vi "Text control 2 v0.5.vi"() -> ()   [LabVIEW 2016]
panel:
  out "error out":errorcluster
  in  "Units":bool
  out "Elapsed Time":dbl caption="Elapsed Time (s)"
  out "Ion vs time":cluster{"Y data in":dbl[], "X data in":dbl[]}[](graph)
  out "Ig":dbl format="%.2e"
  out "Id":dbl format="%.2e"
  out "Is":dbl format="%.2e"
  out "I vs Vg":cluster{"Y data in":dbl[], "X data in":dbl[]}[](graph)
  in  "Panel Controls 2":T1={"Emergency Stop"=refnum, "TransGraph Max"=1e-05, "Text/Graph (text=false)"=TRUE, "TransGraph Min"=1e-11} {"TransGraph Min" format="%.2e"; "TransGraph Max" format="%.2e"}
  out "Currently running:":string="#output s 0 0 0 -0.008 0.008 0.002"
  in  "Lines left to run:":string
  in  "Standby":T2
  in  "Full Reset":bool
  in  "SMU4":cluster{"on/off":bool, "Voltage":dbl} {"Voltage" min=-100.0 max=100.0 format="%.2f"}
  in  "Source/Drain Range":u8(slide)=6 max=11 scale=0.0..11.0
  in  "Source/Drain\nRange mode":u16(ring) items=["Auto", "Limited", "Fixed"]
  in  "Gate Range":u8(slide)=6 max=11 scale=0.0..11.0
  in  "Gate Range\nmode":u16(ring) items=["Auto", "Limited", "Fixed"]
  in  "Gate":T3={"Gate Start"=0.0, "Gate Stop"=2.0, "Gate Step (linear only)"=1.0, "Gate Compliance"=0.0001, "Gate PComp"=0.0, "Range mode"=0, "Range"=6} {"Range" max=11 scale=0.0..11.0; "Range mode" items=["Auto", "Limited", "Fixed"]; "Gate PComp" format="%^.2e"; "Gate Compliance" format="%^.2e"; "Gate Step (linear only)" format="%^.4e"; "Gate Stop" format="%^.4e"; "Gate Start" format="%^.4e"}
  in  "Drain 2":T4={"Drain Start"=0.0, "Drain Stop"=2.0, "Drain Compliance"=0.0001, "Drain Step"=1.0, "Drain PComp"=0.0, "Range mode"=0, "Range"=6} {"Range" max=11 scale=0.0..11.0; "Range mode" items=["Auto", "Limited", "Fixed"]; "Drain PComp" format="%^.2e"; "Drain Step" format="%^.4e"; "Drain Compliance" format="%^.2e"; "Drain Stop" format="%^.4e"; "Drain Start" format="%^.4e"}
  in  "Timings 2":T5={"integration time"=0, "Short/Long integration time"=0.00064, "hold time (sec)"=0.0, "delay time (sec)"=0.0, "Step Time (0 disables)"=0.0, "sweep method"=0, "Pulse period"=0.005, "Base voltage"=0.0, "Pulse width"=0.0005} {"Pulse width" min=0.0005 max=0.1 step=0.0001 format="%.4f"; "Base voltage" format="%^.4e"; "Pulse period" min=0.005 max=1.0 step=0.0001 format="%.4f"; "sweep method" items=["Continuous", "Pulsed"]; "Step Time (0 disables)" format="%.2f"; "delay time (sec)" format="%.4f"; "hold time (sec)" format="%.4f"; "Short/Long integration time" format="%^.0e"; "integration time" scale=0.0..2.0}
  in  "Panel Controls":T6={"Emergency Stop"=refnum, "TransGraph Max"=1e-05, "Text/Graph (text=false)"=TRUE} {"TransGraph Max" format="%.2e"}
  in  "Interrupt run":bool
  in  "Drain: Compliance":dbl=0.001 format="%.8f"
  in  "Gate: Compliance":dbl=0.001 format="%.8f"
  out "Path":path=path "C:/users/rlp38/09Apr2009LTtesting/test2.txt"
  in  "hold time /s":dbl format="%.2f"
  in  "delay time /s":dbl format="%.2f"
  in  "integration time":u32(slide) max=2 step=1 scale=0.0..2.0
  in  "Integration time (short)":dbl=0.0019 min=8e-05 max=0.0019 step=8e-05 format="%^.0e"
  in  "Integration time (long)":dbl=0.32 min=0.04 max=2.0 step=0.02 format="%.2f"
  in  "Step delay /s":dbl format="%.2f"
  in  "Program":string="#pulsedstressV d 0.03 20 0 0.5 0.0827 5\n#\nitime s\ngaterangemode l\ndrainrangemode l\n#pulsed on 0.05 0 0.02\ntransfer d 1 -1 -0.1 -1 -1 0\nwait-min 1\ntransfer d 1 -1 -0.1 -1 -1 0\n#transfer d -10 40 1 5 40 35\n#transfer d -10 40 1 5 40 35\n#output d 0 40 20 0 40 1\n#\n#\n#sample 1 0.008 221 6 0.003\n#samplei 400e-6 200 6 0.002 0.1\n#vsu2pulse -10 4\n#\n#stressV 0.016 0.03 2e-4 0.1e-3 11\n#stressI 220e-7 0.08 15\n#transfer s -1 1 0.5 -0.005 0.005 0.005\n#output s 0 0 0 -0.008 0.008 0.002\n"
  # "Syntax:\nitime [s|m|l]\ngaterangemode [a|l|f]\ndrainrangemode [a|l|f]\npulsed [on|off] PulsePeriod(sec) PulseBaseVoltage PulseONWidth(sec)\nstandby [on l off]\nwait NumMilliseconds\nwait-min NumMinutes\n# texthere = comment\ntransfer [s|d] VgStart VgStop VgStep VdStart VdStop VdStep\noutput [s|d] VgStart VgStop VgStep VdStart VdStop VdStep\nsample Vg Vd NumSamples Time(s) SampleInterval(s)\nsamplei Idg NumSamples Time(s) SampleInterval(s) VDGcompliance\n# if in doubt use SampleInterval(s) = 0.004\nstressV VG VD IGcompliance IDcompliance Duration(sec)\nstressI IDG VDGcompliance Duration(sec)\nvsu2pulse Bias Duration(s)\npulsedstressV [s|d] VEstop VgON VgOFF Period(s) PulseONwidth(s) Vd\nsample-fpp Vg Vd NumSamples Time\nresample-fpp Vg Vd\ntransfer-fpp [s|d] VgStart VgStop VgStep VdStart VdStop VdStep\noutput-fpp [s|d] VgStart VgStop VgStep VdStart VdStop VdStep"
  # "Sec"
  # "Min"
  # "Original Filename (.txt is removed)-Prefix-ElapsedTime (in sec)-Suffix (must include .txt)"
  # "100 samples is approx 13s with medium integration"
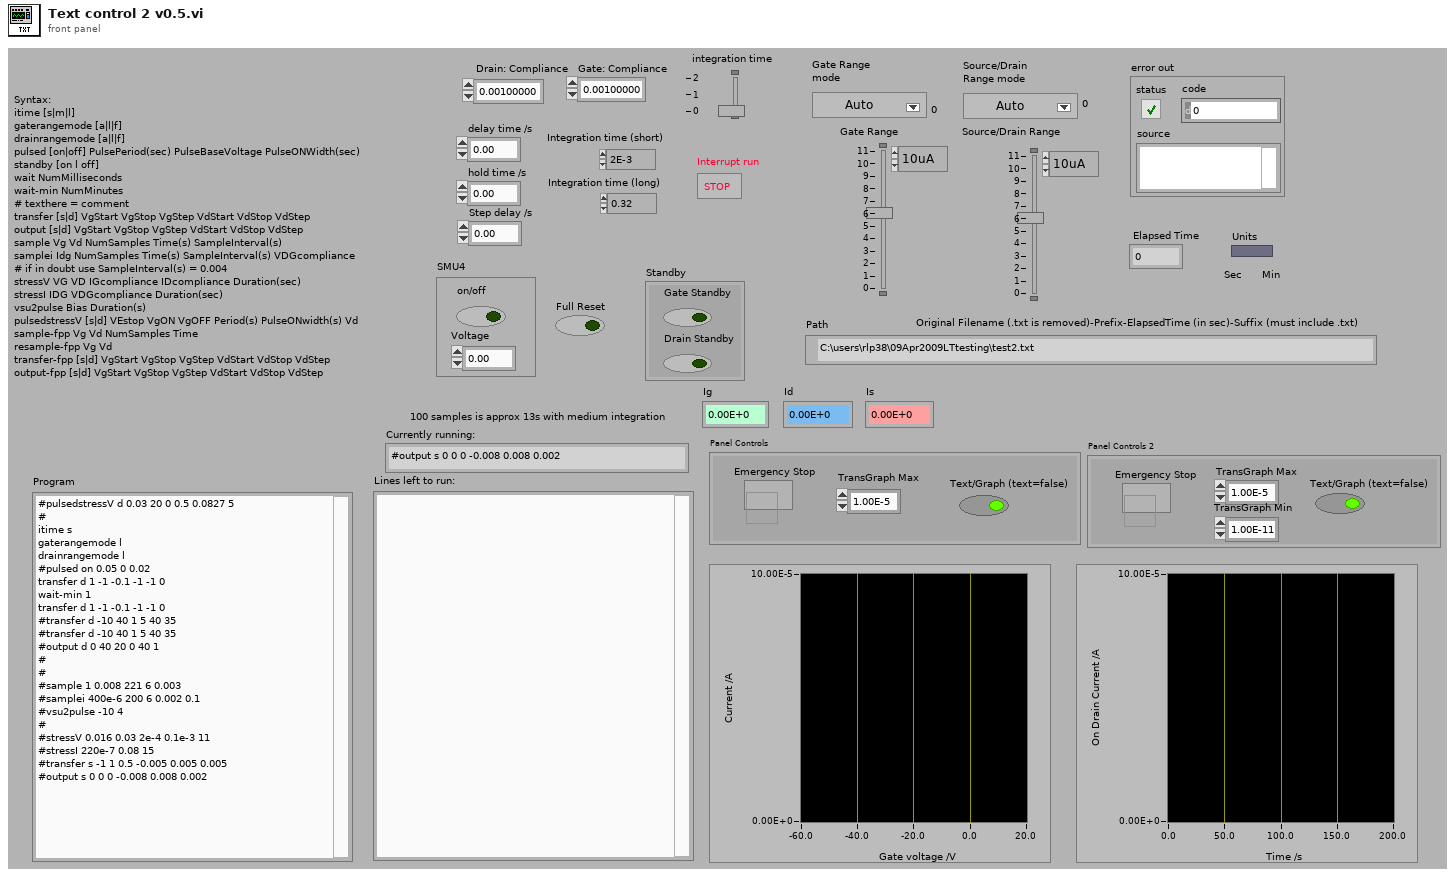
[diagram p1: front panel]
types:
  T1 = cluster{"Emergency Stop":refnum<vi>, "TransGraph Max":dbl, "Text/Graph (text=false)":bool, "TransGraph Min":dbl}
  T2 = cluster{"Gate Standby":bool, "Drain Standby":bool}
  T3 = cluster{"Gate Start":dbl, "Gate Stop":dbl, "Gate Step (linear only)":dbl, "Gate Compliance":dbl, "Gate PComp":dbl, "Range mode":u16, "Range":u8}
  T4 = cluster{"Drain Start":dbl, "Drain Stop":dbl, "Drain Compliance":dbl, "Drain Step":dbl, "Drain PComp":dbl, "Range mode":u16, "Range":u8}
  T5 = cluster{"integration time":u32, "Short/Long integration time":dbl, "hold time (sec)":dbl, "delay time (sec)":dbl, "Step Time (0 disables)":dbl, "sweep method":u16, "Pulse period":dbl, "Base voltage":dbl, "Pulse width":dbl}
  T6 = cluster{"Emergency Stop":refnum<vi>, "TransGraph Max":dbl, "Text/Graph (text=false)":bool}
  T7 = enum16{"open", "replace", "create", "open or create", "replace or create", "replace or create with confirmation"}
  T8 = cluster{"V2 Start":dbl, "V2 Step":dbl, "Number of points":i32}
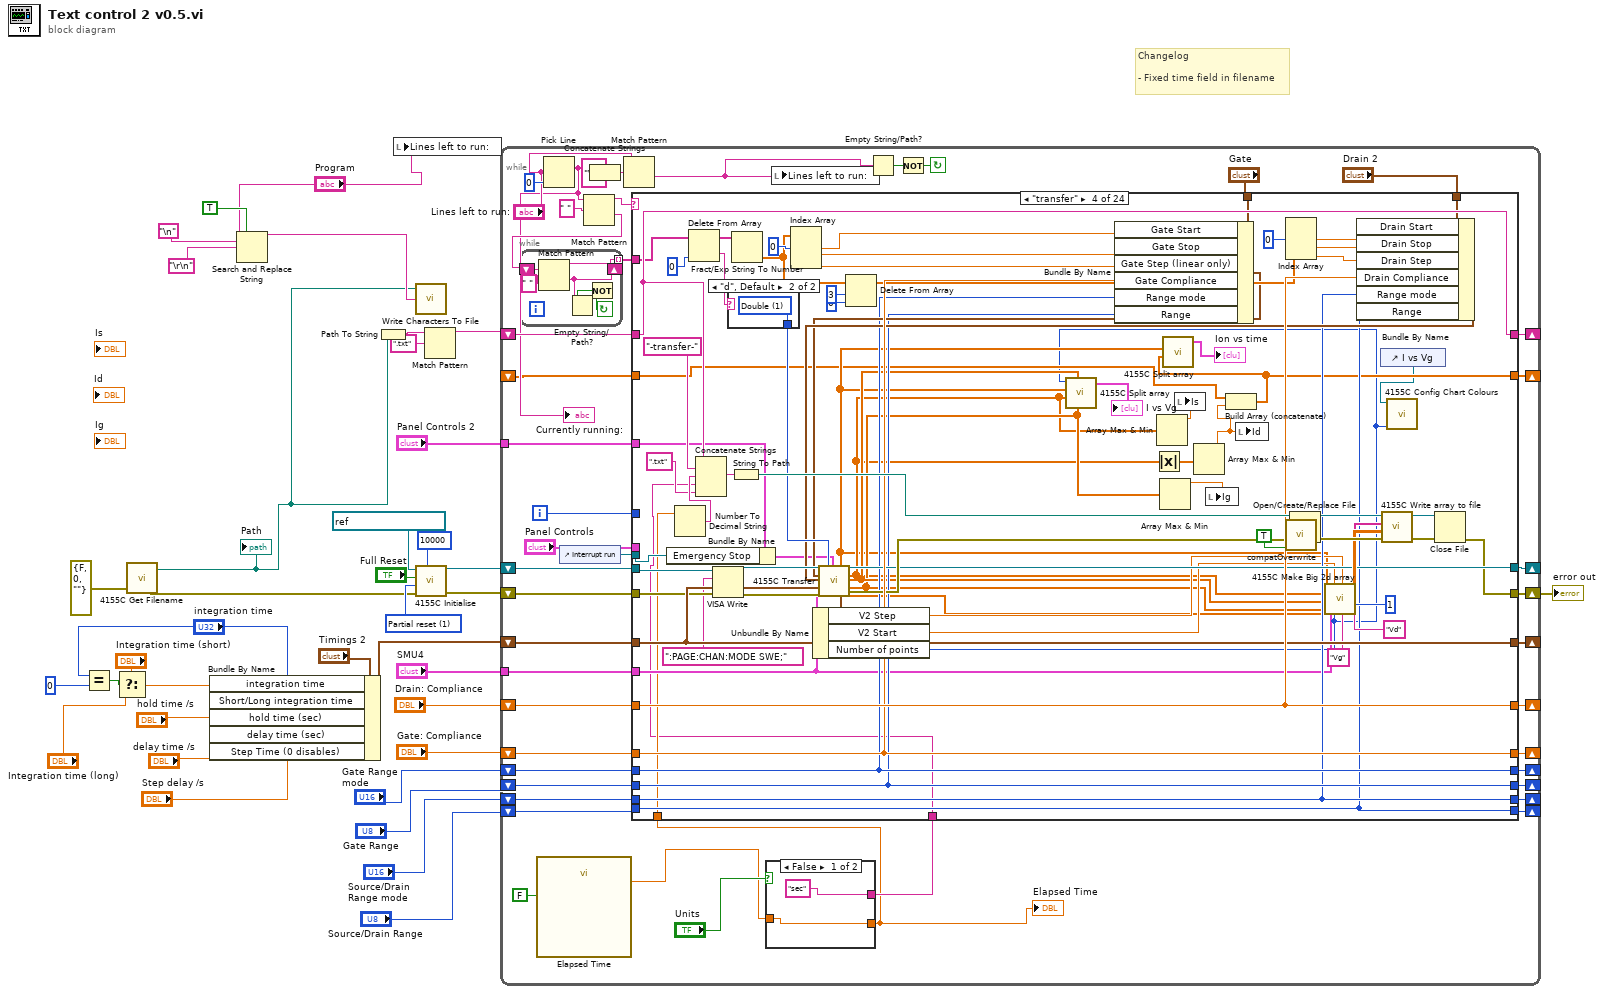
[diagram p0: block diagram]
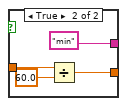
[diagram p2: hidden frame]
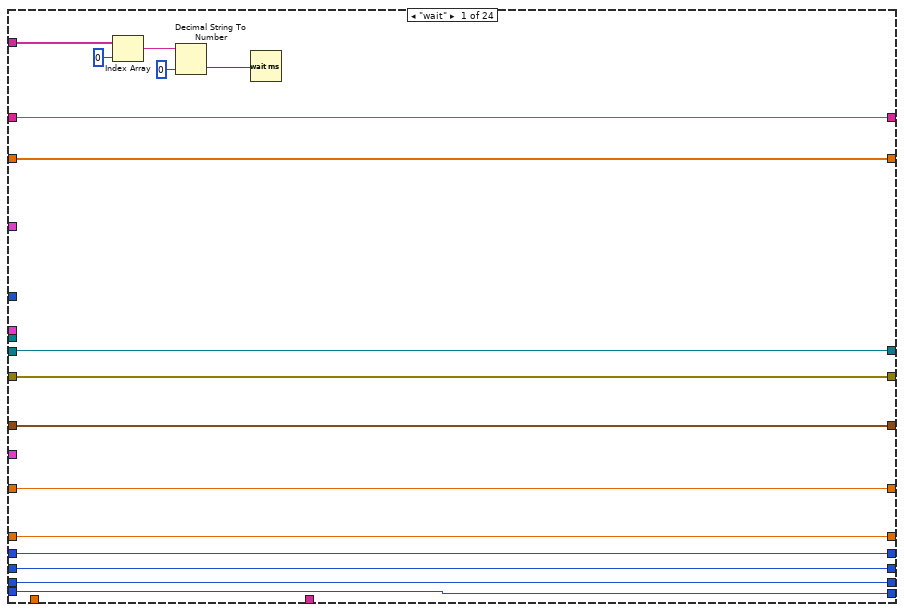
[diagram p3: hidden frame]
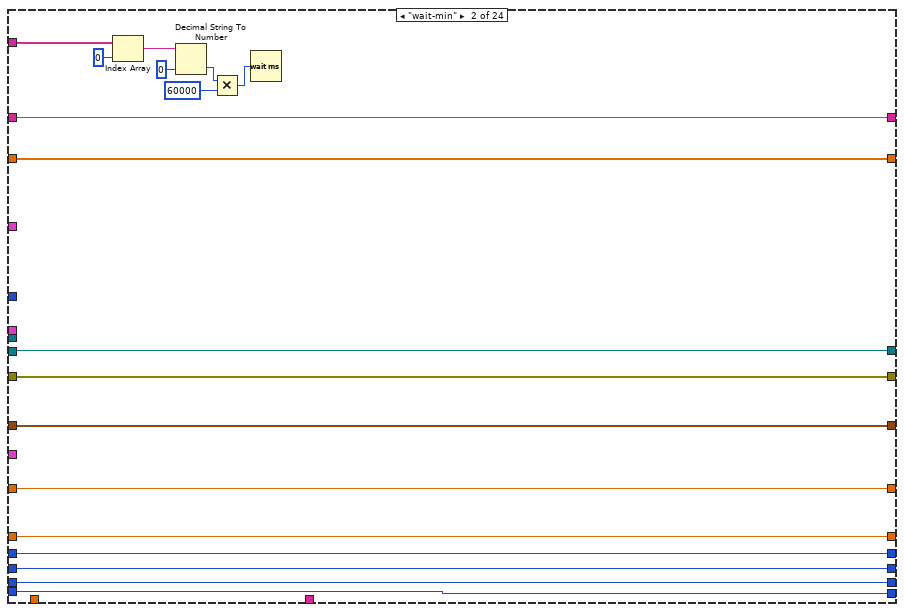
[diagram p4: hidden frame]
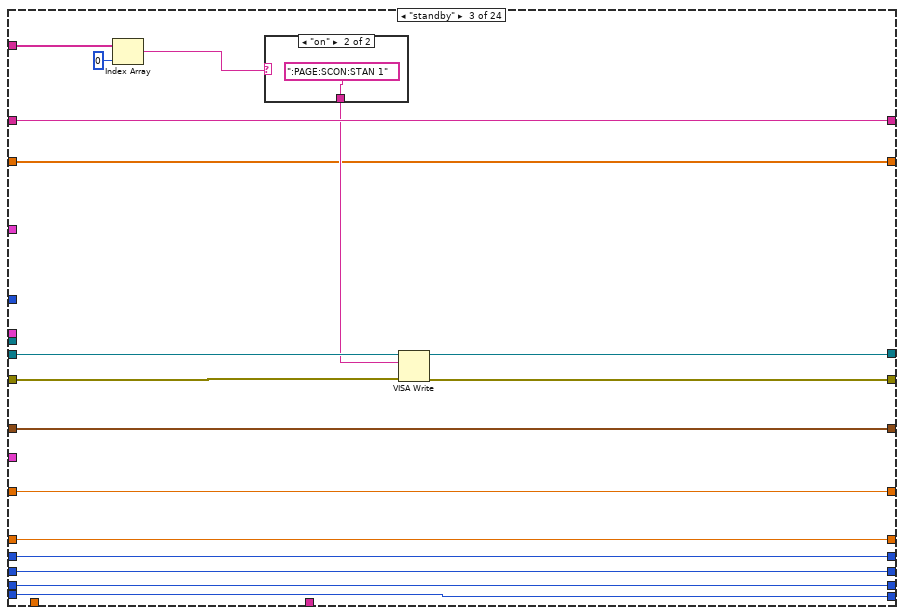
[diagram p5: hidden frame]
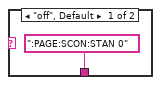
[diagram p6: hidden frame]
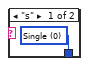
[diagram p7: hidden frame]
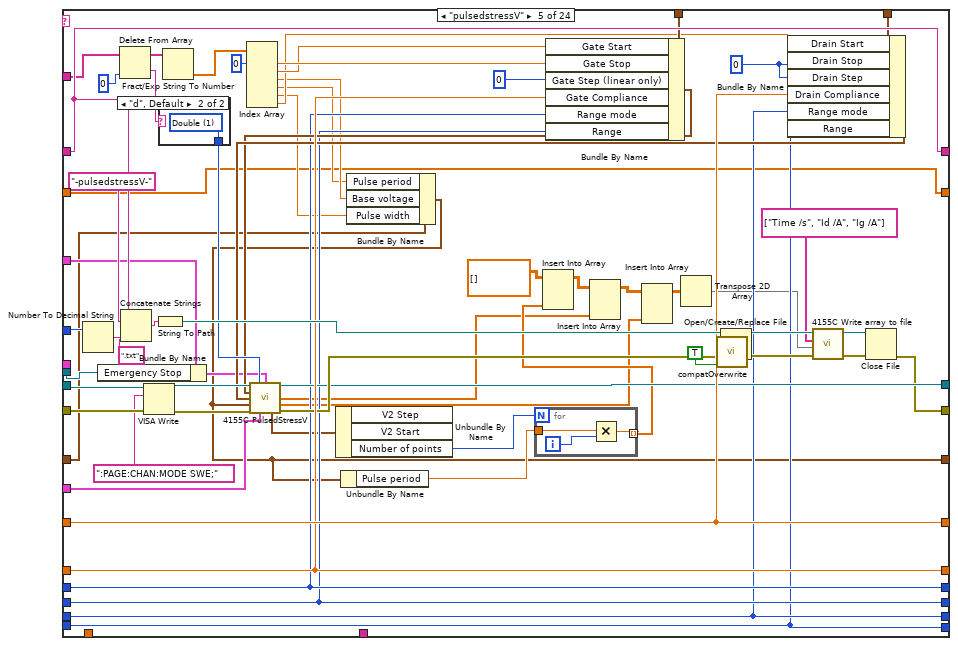
[diagram p8: hidden frame]
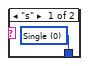
[diagram p9: hidden frame]
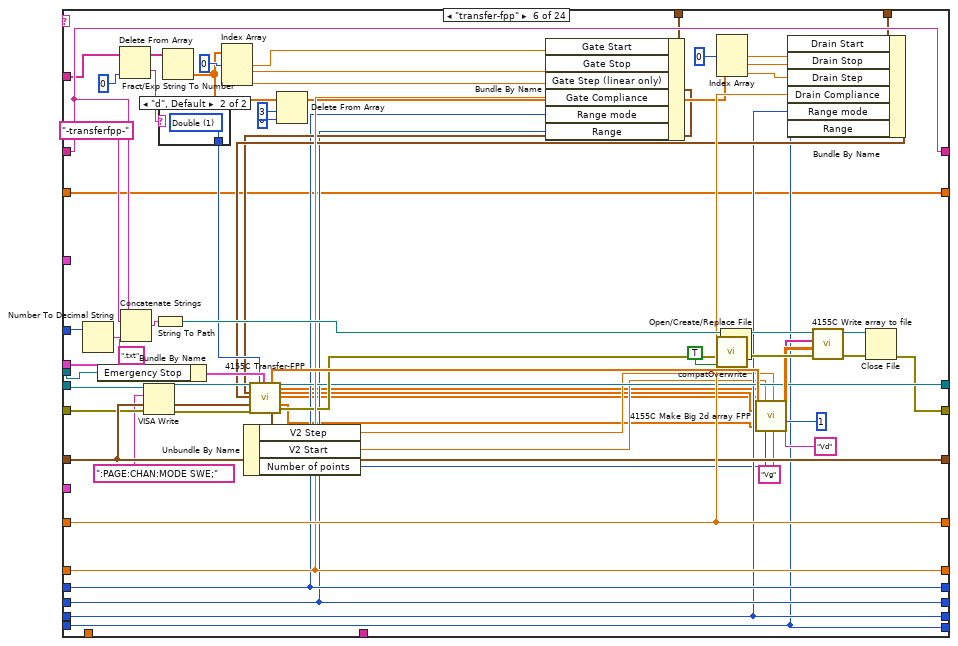
[diagram p10: hidden frame]
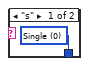
[diagram p11: hidden frame]
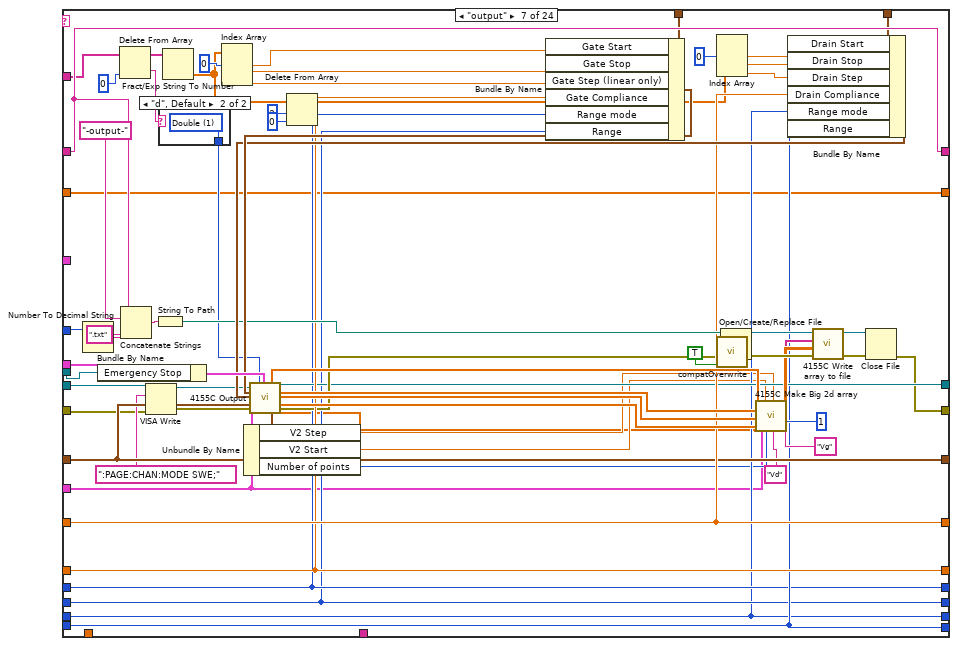
[diagram p12: hidden frame]
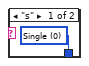
[diagram p13: hidden frame]
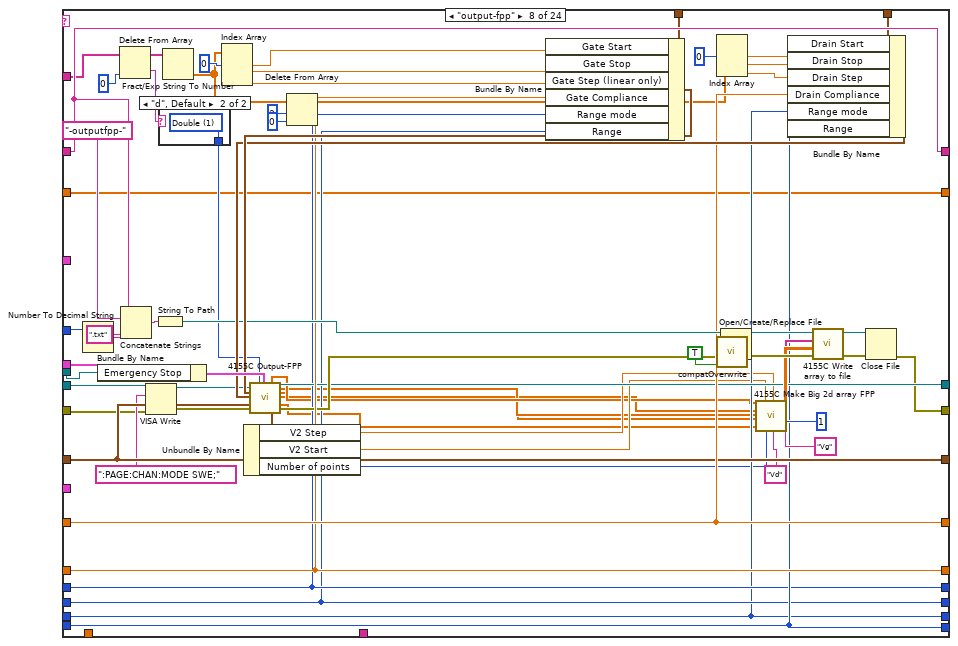
[diagram p14: hidden frame]
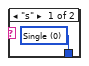
[diagram p15: hidden frame]
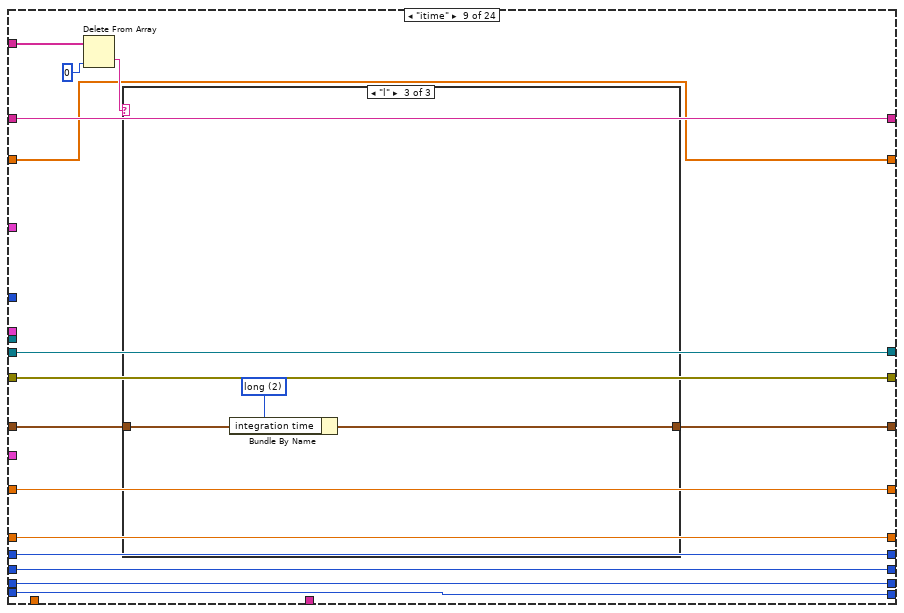
[diagram p16: hidden frame]
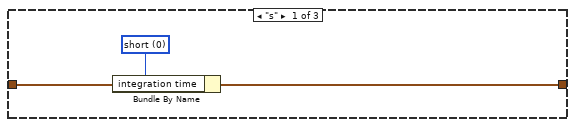
[diagram p17: hidden frame]
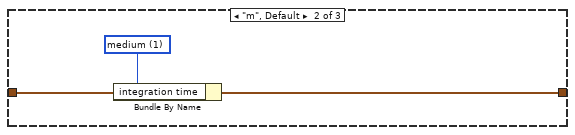
[diagram p18: hidden frame]
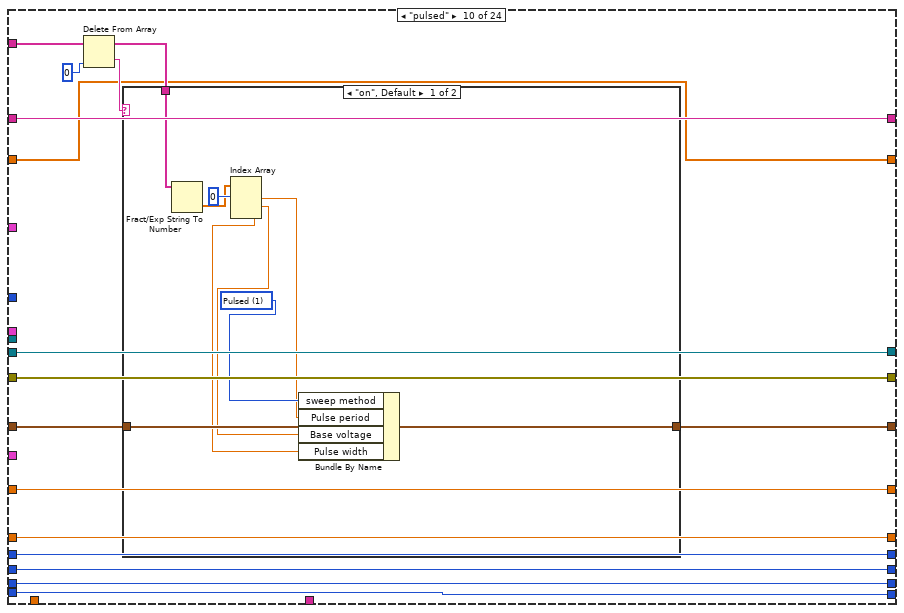
[diagram p19: hidden frame]
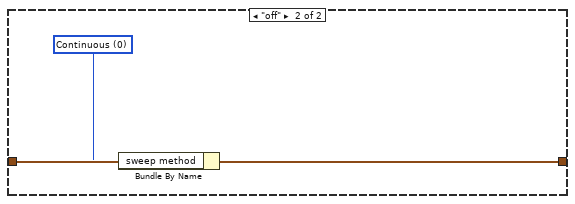
[diagram p20: hidden frame]
diagram:
  w28 = u16 1 items=["Reset All", "Partial reset"] ("Type of reset")
  # "Changelog\n\n- Fixed time field in filename"
  n1 = Equal?(x="integration time", y=u32 0) -> (x = y?=w32:bool)
  n2 = Select(t="Integration time (short)", s=w32, f="Integration time (long)") -> (s? t:f=w36:dbl)
  n3 = call <userlib>:"4155C Get Filename.vi"("error in (no error)"=errorcluster {"status"=FALSE, "code"=0, "source"=""}) -> ("error out"=w23:errorcluster, "path"=w7:path)  [unwired: 2 in, 1 out]
  "Path" <- w7
  n4 = Bundle By Name(cluster="Timings 2", "integration time"="integration time", "Short/Long integration time"=w36, "hold time (sec)"="hold time /s", "delay time (sec)"="delay time /s", "Step Time (0 disables)"="Step delay /s") -> (w20:T5)
  n5 = Search and Replace String(replace all?=TRUE ("replace all? (F)"), input string="Program", search string="\n", replace string="\r\n") -> (result string=w10:string)  [unwired: 4 in, 3 out]
  n6 = Path To String(path=w7) -> (string=w6:string)
  n7 = local write "Lines left to run:"("Program") -> ()
  n8 = call <vilib>:"Write Characters To File.vi"("character string"=w10, "file path (dialog if empty)"=w7) -> ()  [unwired: 3 in, 1 out]
  n9 = call <userlib>:"4155C Initialise.vi"("VISA resource name in"=refnum<visa-resource-name> "GPIB0::14::INSTR", "Reset"="Full Reset", "Type of reset"=w28, "error in (no error)"=w23, "VISA Timeout Value"=u32 10000) -> ("VISA Resource Name out"=w22:refnum<visa-resource-name>, "error out"=w21:errorcluster)
  n10 = Match Pattern(string=w6, regular expression=".txt") -> (before substring=w5:string)  [unwired: 1 in, 3 out]
  n11 = while {
    tunnel: "SMU4" -> [w49]
    shift-left: "Source/Drain Range" -> [w54]
    shift-right: [w50] -> _
    shift-left: "Source/Drain\nRange mode" -> [w55]
    shift-right: [w51] -> _
    shift-left: "Gate Range" -> [w56]
    shift-right: [w52] -> _
    shift-left: "Gate Range\nmode" -> [w57]
    shift-right: [w53] -> _
    shift-left: "Gate: Compliance" -> [w69]
    shift-right: [w63] -> _
    shift-left: "Drain: Compliance" -> [w70]
    shift-right: [w64] -> _
    shift-left: w20 -> [w71]
    shift-right: [w65] -> _
    shift-left: w21 -> [w72]
    shift-right: [w66] -> w1
    shift-left: w22 -> [w73]
    shift-right: [w67] -> _
    shift-left: w5 -> [w74]
    shift-right: [w62] -> _
    tunnel: "Panel Controls 2" -> [w45]
    shift-right: [w44] -> _
    shift-left: _ -> [w43]
    i -> [w68]
    stop <- w82 continue-if-true
    n12 = call "Elapsed Time"("Auto Reset"=FALSE) -> ("Elapsed Time (s)"=w39:dbl)  [unwired: 11 in, 7 out]
    n13 = Pick Line(multi-line string="Lines left to run:", line index=0) -> (output string=w46:string)  [unwired: 1 in]
    "Currently running:" <- w46
    n14 = control-ref of="Interrupt run"() -> (w61:refnum<vi>)
    n15 = Match Pattern(string=w46, regular expression=" ") -> (before substring=w77:string, after substring=w76:string)  [unwired: 1 in, 2 out]
    n16 = while {
      tunnel: [w90] -> w75 mode=indexing
      shift-left: w76 -> [w92]
      shift-right: [w91] -> _
      stop <- w94 continue-if-true
      n17 = Match Pattern(string=w92, regular expression=" ") -> (before substring=w90:string, after substring=w91:string)  [unwired: 1 in, 2 out]
      n18 = Empty String/Path?(string/path=w91) -> (empty?=w95:bool)
      n19 = Not(x=w95) -> (.not. x?=w94:bool)
    }
    n20 = Concatenate Strings(w46, "\n" ("Substring")) -> (w80:string)
    n21 = Match Pattern(string="Lines left to run:", regular expression=w80) -> (after substring=w47:string)  [unwired: 1 in, 3 out]
    n22 = case shown="False" "Units" {
      tunnel: ["sec" "min"] -> w40
      tunnel: [w84 w88] -> w38
      tunnel: w39 -> [w84 w87]
      frame False {
      }
      frame True {
        n23 = Divide(x=w87, y=60.0) -> (x/y=w88:dbl)
      }
    }
    "Elapsed Time" <- w38
    n24 = case shown="\"transfer\"" w77 {
      tunnel: w75 -> [w111 w129 w146 w207 w275 w342 w407 w480 w518 w543 w569 w593 w613 w626 _ _ w724 w783 _ w845 w887 w927 w995 w1055]
      tunnel: w74 -> [w106 w125 w144 w215 w282 w350 w415 w488 w507 w532 w561 w586 w607 w619 w637 w676 w702 w765 w796 w832 w874 w915 w989 w1051]
      tunnel: w73 -> [w105 w124 w135 w185 w266 w319 w383 w456 w508 w533 w562 w587 w608 w620 w642 w679 w731 w790 w800 w852 w894 w934 w1002 w1008]
      tunnel: w72 -> [w104 w123 w134 w184 w265 w318 w380 w453 w509 w534 w563 w588 w609 w621 w641 w648 w730 w789 w799 w851 w893 w933 w1001 w1007]
      tunnel: w71 -> [w103 w122 w143 w211 w240 w346 w411 w484 w517 w542 w560 w585 w606 w618 w640 w672 w693 w757 w805 w825 w867 w908 w988 w1050]
      tunnel: w70 -> [w102 w121 w142 w213 w280 w348 w413 w486 w516 w541 w568 w592 w612 w625 w639 w657 w729 w788 w808 w850 w892 w932 w1000 w1060]
      tunnel: w69 -> [w101 w120 w141 w212 w279 w347 w412 w485 w515 w540 w567 w591 w611 w624 w638 w658 w703 w766 w807 w833 w875 w916 w990 w1052]
      tunnel: w68 -> [_ _ _ _ w283 w351 w416 w489 _ _ _ _ _ _ _ w674 w728 w787 _ w849 w891 w931 w999 w1059]
      tunnel: [w105 w124 w133 w209 w277 w344 w409 w482 w508 w533 w562 w587 w608 w620 w642 w679 w694 w738 w798 w826 w868 w909 w940 w1010] -> w67
      tunnel: [w104 w123 w132 w208 w276 w343 w408 w481 w509 w534 w563 w588 w609 w621 w641 w647 w704 w739 w797 w834 w876 w917 w939 w1009] -> w66
      tunnel: [w103 w122 w143 w211 w236 w346 w411 w484 w510 w535 w560 w585 w606 w618 w640 w672 w693 w757 w805 w825 w867 w908 w988 w1050] -> w65
      tunnel: [w102 w121 w142 w213 w280 w348 w413 w486 w516 w541 w568 w592 w612 w625 w639 w657 w729 w788 w808 w850 w892 w932 w1000 w1060] -> w64
      tunnel: [w101 w120 w141 w212 w279 w347 w412 w485 w515 w540 w567 w591 w611 w624 w638 w658 w703 w766 w807 w833 w875 w916 w990 w1052] -> w63
      tunnel: [w106 w125 w144 w215 w282 w350 w415 w488 w507 w532 w561 w586 w607 w619 w637 w676 w702 w765 w796 w832 w874 w915 w989 w1051] -> w62
      tunnel: w61 -> [_ _ _ w218 w287 w356 w424 w493 _ _ _ _ _ _ _ _ w699 w762 _ w831 w873 w914 w960 w1026]
      tunnel: "Gate" -> [_ _ _ w194 w269 w329 w394 w467 _ _ _ _ _ _ _ _ _ _ _ _ _ _ _ _]
      tunnel: "Drain 2" -> [_ _ _ w193 w268 w328 w393 w466 _ _ _ _ _ _ _ _ _ _ _ _ _ _ _ _]
      tunnel: "Panel Controls" -> [_ _ _ _ _ w327 w392 w465 _ _ _ _ _ _ _ _ _ _ _ _ _ _ _ _]
      tunnel: w57 -> [w100 w119 w140 w178 w259 w312 w378 w451 w514 w539 _ w584 w605 w617 w636 w659 w689 w753 w801 w821 w863 w904 w984 w1046]
      tunnel: w56 -> [w99 w118 w139 w177 w258 w311 w377 w450 w513 w538 w566 _ w596 w623 w635 w660 w690 w754 w802 w822 w864 w905 w985 w1047]
      tunnel: w55 -> [w98 w117 w138 w176 w257 w310 w376 w449 w512 w537 w565 w590 w610 _ w634 w661 w691 w755 w803 w823 w865 w906 w986 w1048]
      tunnel: w54 -> [w97 w116 w137 w175 w256 w309 w379 w452 w511 w536 w564 w589 _ w622 w633 w662 w692 w756 w804 w824 w866 w907 w987 w1049]
      tunnel: [w100 w119 w140 w178 w259 w312 w378 w451 w514 w539 w559 w584 w605 w617 w636 w659 w689 w753 w801 w821 w863 w904 w984 w1046] -> w53
      tunnel: [w99 w118 w139 w177 w258 w311 w377 w450 w513 w538 w566 w576 w596 w623 w635 w660 w690 w754 w802 w822 w864 w905 w985 w1047] -> w52
      tunnel: [w98 w117 w138 w176 w257 w310 w376 w449 w512 w537 w565 w590 w610 w616 w634 w661 w691 w755 w803 w823 w865 w906 w986 w1048] -> w51
      tunnel: [w97 w116 w137 w175 w256 w309 w379 w452 w511 w536 w564 w589 w597 w622 w633 w662 w692 w756 w804 w824 w866 w907 w987 w1049] -> w50
      tunnel: w49 -> [_ _ _ w170 w252 _ w370 _ _ _ _ _ _ _ _ _ _ _ _ _ _ _ _ _]
      tunnel: w45 -> [_ _ _ w168 w251 _ _ _ _ _ _ _ _ _ _ _ _ _ _ _ _ _ _ _]
      tunnel: [w96 w112 w130 w157 w228 w298 w367 w437 w506 w530 w558 w575 w595 w615 w632 w643 w680 w736 w795 w809 w855 w897 w937 w1003] -> w44
      tunnel: w43 -> [w96 w112 w130 w156 w228 w298 w367 w437 w506 w530 w558 w575 w595 w615 w632 w643 w680 w736 w795 w809 w855 w897 w937 w1003]
      tunnel: w38 -> [_ _ _ w152 _ _ _ _ _ _ _ _ _ _ _ _ _ _ _ _ _ _ _ _]
      tunnel: w40 -> [_ _ _ w149 _ _ _ _ _ _ _ _ _ _ _ _ _ _ _ _ _ _ _ _]
      frame "wait" {
        n25 = Index Array(array=w111, index=0 ("Index")) -> (element=w109:string)
        n26 = Decimal String To Number(string=w109, default (0L)=u32 0) -> (number=w108:u32)  [unwired: 1 in, 1 out]
        n27 = Wait (ms)(milliseconds to wait=w108) -> ()  [unwired: 1 out]
      }
      frame "wait-min" {
        n28 = Index Array(array=w129, index=0 ("Index")) -> (element=w127:string)
        n29 = Decimal String To Number(string=w127, default (0L)=u32 0) -> (number=w115:u32)  [unwired: 1 in, 1 out]
        n30 = Multiply(x=w115, y=u32 60000) -> (x*y=w114:u32)
        n31 = Wait (ms)(milliseconds to wait=w114) -> ()  [unwired: 1 out]
      }
      frame "standby" {
        n32 = Index Array(array=w146, index=0 ("Index")) -> (element=w136:string)
        n33 = case shown="\"on\"" w136 {
          tunnel: [":PAGE:SCON:STAN 0" ":PAGE:SCON:STAN 1"] -> w131
          frame "off", Default {
          }
          frame "on" {
          }
        }
        n34 = VISA Write(VISA resource name=w135, write buffer=w131, error in (no error)=w134) -> (VISA resource name out=w133:refnum<visa-resource-name>, error out=w132:errorcluster)  [unwired: 1 out]
      }
      frame "transfer" {
        n35 = Bundle By Name(cluster=w168, "Emergency Stop"=w218) -> (w169:T1)
        n36 = Number To Decimal String(number=w152) -> (decimal integer string=w151:string)  [unwired: 1 in]
        n37 = Delete From Array(array=w207, index=0 ("Index")) -> (deleted portion=w205:string, array with subset deleted=w204:string[])  [unwired: 1 in]
        n38 = Concatenate Strings(w215, "-transfer-" ("Prefix"), w151, w149, ".txt" ("Suffix")) -> (w217:string)
        n39 = VISA Write(VISA resource name=w185, write buffer=":PAGE:CHAN:MODE SWE;" ("write buffer (\"\")"), error in (no error)=w184) -> (VISA resource name out=w182:refnum<visa-resource-name>, error out=w183:errorcluster)  [unwired: 1 out]
        n40 = case shown="\"d\", Default" w205 {
          tunnel: [w226 w227] -> w203
          frame "s" {
            w226 = u16 0 items=["Single", "Double"] ("sweep mode")
          }
          frame "d", Default {
            w227 = u16 1 items=["Single", "Double"] ("sweep mode")
          }
        }
        n41 = String To Path(string=w217) -> (path=w214:path)
        n42 = Fract/Exp String To Number(string=w204) -> (number=w189:dbl[])  [unwired: 3 in, 1 out]
        n43 = Index Array(array=w189, index #1=0 ("Index")) -> (element #1=w202:dbl, element #2=w201:dbl, element #3=w200:dbl)  [unwired: 2 in]
        n44 = Delete From Array(array=w189, length=3 ("Length"), index=0 ("Index")) -> (array with subset deleted=w187:dbl[])  [unwired: 1 out]
        n45 = Bundle By Name(cluster=w194, "Gate Start"=w202, "Gate Stop"=w201, "Gate Step (linear only)"=w200, "Gate Compliance"=w212, "Range mode"=w178, "Range"=w177) -> (w179:T3)
        n46 = Index Array(array=w187, index #1=0 ("Index")) -> (element #1=w197:dbl, element #2=w196:dbl, element #3=w195:dbl)  [unwired: 2 in]
        n47 = call <vilib>:"compatOverwrite.vi"("overwrite (F)"=TRUE) -> ("overwrite?"=w167:T7)
        n48 = Bundle By Name(cluster=w193, "Drain Start"=w197, "Drain Stop"=w196, "Drain Step"=w195, "Drain Compliance"=w213, "Range mode"=w176, "Range"=w175) -> (w180:T4)
        n49 = call <userlib>:"4155C Transfer.vi"("VISA resource name in"=w182, "Gate"=w179, "Drain"=w180, "Timings"=w211, "error in (no error)"=w183, "SMU4"=w170, "sweep mode"=w203, "Panel Controls"=w169) -> ("VG"=w158:dbl[], "Outparams"=w174:T8, "VISA Resource Name out"=w209:refnum<visa-resource-name>, "IS"=w160:dbl[], "ID"=w165:dbl[], "IG"=w161:dbl[], "error out"=w210:errorcluster, "SMU4"=w171:dbl[])  [unwired: 12 in]
        n50 = Unbundle By Name(w174) -> ("V2 Step"=w173:dbl, "V2 Start"=w172:dbl, "Number of points"=w154:i32)
        n51 = call <userlib>:"4155C Split array.vi"("Number of VAR2 steps"=w154, "Y2 data in"=w165, "X data in"=w158, "Y1 data in"=w160, "Y3 data in"=w161) -> ("Array of clusters"=→"I vs Vg":cluster{"Y data in":dbl[], "X data in":dbl[]}[])  [unwired: 2 in, 1 out]
        n52 = Absolute Value(x=w160) -> (abs(x)=w164:dbl[])
        n53 = Array Max & Min(array=w160) -> (max value=w162:dbl)  [unwired: 3 out]
        n54 = Array Max & Min(array=w161) -> (max value=w163:dbl)  [unwired: 3 out]
        n55 = local write "Is"(w162) -> ()
        n56 = Array Max & Min(array=w164) -> (max value=w155:dbl)  [unwired: 3 out]
        n57 = local write "Ig"(w163) -> ()
        n58 = Build Array (concatenate)(w156, w155) -> (w157:dbl[])
        n59 = call <userlib>:"4155C Split array.vi"("X data in"=w158, "Y1 data in"=w157) -> ("Array of clusters"=→"Ion vs time":cluster{"Y data in":dbl[], "X data in":dbl[]}[])  [unwired: 5 in, 1 out]
        n60 = local write "Id"(w155) -> ()
        n61 = Open/Create/Replace File(file path (use dialog)=w214, error in=w210, operation (0:open)=w167) -> (refnum out=w223:refnum<file>, error out=w224:errorcluster)  [unwired: 3 in, 1 out]
        n62 = call <userlib>:"4155C Make Big 2d array.vi"("1D Var1"=w158, "1d IS"=w160, "1d ID"=w165, "1d IG"=w161, "1d SMU4"=w171, "SMU4"=w170, "VAR2 START"=w172, "Number of VAR2 steps"=w154, "VAR2 STEP"=w173, "VAR1 Name"="Vg", "Decimal places in header"=i8 1, "VAR2 Name"="Vd") -> ("Header array"=w219:string[], "Data array"=w220:dbl[][])  [unwired: 14 in]
        n63 = control-ref of="I vs Vg"() -> (w153:refnum<vi>)
        n64 = call <userlib>:"4155C Write array to file.vi"("Byte Stream File Refnum"=w223, "Header"=w219, "Data Array"=w220, "error in (no error)"=w224) -> ("dup refnum"=w221:refnum<file>, "error out"=w222:errorcluster)  [unwired: 1 in]
        n65 = call <userlib>:"4155C Config Chart Colours.vi"("Numeric"=w154, "XY Graph 2"=w153) -> ()  [unwired: 6 in]
        n66 = Close File(refnum=w221, error in=w222) -> (error out=w208:errorcluster)  [unwired: 1 out]
      }
      frame "pulsedstressV" {
        w234 = 0
        n67 = Number To Decimal String(number=w283) -> (decimal integer string=w284:string)  [unwired: 1 in]
        n68 = Bundle By Name(cluster=w251, "Emergency Stop"=w287) -> (w253:T1)
        n69 = Delete From Array(array=w275, index=0 ("Index")) -> (deleted portion=w273:string, array with subset deleted=w272:string[])  [unwired: 1 in]
        n70 = Concatenate Strings(w282, "-pulsedstressV-" ("Substring"), w284, ".txt" ("Substring")) -> (w286:string)
        n71 = VISA Write(VISA resource name=w266, write buffer=":PAGE:CHAN:MODE SWE;" ("write buffer (\"\")"), error in (no error)=w265) -> (VISA resource name out=w263:refnum<visa-resource-name>, error out=w264:errorcluster)  [unwired: 1 out]
        n72 = String To Path(string=w286) -> (path=w281:path)
        n73 = case shown="\"d\", Default" w273 {
          tunnel: [w296 w297] -> w271
          frame "s" {
            w296 = u16 0 items=["Single", "Double"] ("sweep mode")
          }
          frame "d", Default {
            w297 = u16 1 items=["Single", "Double"] ("sweep mode")
          }
        }
        n74 = Fract/Exp String To Number(string=w272) -> (number=w267:dbl[])  [unwired: 3 in, 1 out]
        n75 = Index Array(array=w267, index #1=0 ("Index")) -> (element #1=w243:dbl, element #2=w242:dbl, element #3=w239:dbl, element #4=w238:dbl, element #5=w237:dbl, element #6=w241:dbl)  [unwired: 5 in]
        n76 = Bundle By Name(cluster=w240, "Pulse period"=w238, "Base voltage"=w239, "Pulse width"=w237) -> (w236:T5)
        n77 = Unbundle By Name(w236) -> ("Pulse period"=w244:dbl)
        n78 = Bundle By Name(cluster=w269, "Gate Start"=w242, "Gate Stop"=w243, "Gate Step (linear only)"=0, "Gate Compliance"=w279, "Range mode"=w259, "Range"=w258) -> (w260:T3)
        n79 = call <vilib>:"compatOverwrite.vi"("overwrite (F)"=TRUE) -> ("overwrite?"=w229:T7)
        n80 = Bundle By Name(cluster=w268, "Drain Start"=w241, "Drain Stop"=w234, "Drain Step"=w234, "Drain Compliance"=w280, "Range mode"=w257, "Range"=w256) -> (w261:T4)
        n81 = call <userlib>:"4155C PulsedStressV.vi"("VISA resource name in"=w263, "sweep mode"=w271, "Panel Controls"=w253, "Gate"=w260, "Drain"=w261, "Timings"=w236, "error in (no error)"=w264, "SMU4"=w252) -> ("VISA Resource Name out"=w277:refnum<visa-resource-name>, "ID"=w232:dbl[], "IG"=w230:dbl[], "Outparams"=w254:T8, "error out"=w278:errorcluster)  [unwired: 3 in]
        n82 = Unbundle By Name(w254) -> ("Number of points"=w231:i32)  [unwired: 2 out]
        n83 = for {
          N: w231 -> [_]
          tunnel: [w293] -> w233 mode=indexing
          tunnel: w244 -> [w295]
          i -> [w294]
          n84 = Multiply(x=w295, y=w294) -> (x*y=w293:dbl)
        }
        n85 = Insert Into Array(array=dbl[][] [] ("Input Array"), new element=w233) -> (w245:dbl[][])  [unwired: 2 in]
        n86 = Insert Into Array(array=w245, new element=w232) -> (w250:dbl[][])  [unwired: 2 in]
        n87 = Insert Into Array(array=w250, new element=w230) -> (w249:dbl[][])  [unwired: 2 in]
        n88 = Transpose 2D Array(2D array=w249) -> (transposed array=w248:dbl[][])
        n89 = Open/Create/Replace File(file path (use dialog)=w281, error in=w278, operation (0:open)=w229) -> (refnum out=w290:refnum<file>, error out=w291:errorcluster)  [unwired: 3 in, 1 out]
        n90 = call <userlib>:"4155C Write array to file.vi"("Byte Stream File Refnum"=w290, "Header"=string[] ["Time /s", "Id /A", "Ig /A"], "Data Array"=w248, "error in (no error)"=w291) -> ("dup refnum"=w288:refnum<file>, "error out"=w289:errorcluster)  [unwired: 1 in]
        n91 = Close File(refnum=w288, error in=w289) -> (error out=w276:errorcluster)  [unwired: 1 out]
      }
      frame "transfer-fpp" {
        n92 = Number To Decimal String(number=w351) -> (decimal integer string=w352:string)  [unwired: 1 in]
        n93 = Bundle By Name(cluster=w327, "Emergency Stop"=w356) -> (w364:T6)
        n94 = Delete From Array(array=w342, index=0 ("Index")) -> (deleted portion=w340:string, array with subset deleted=w339:string[])  [unwired: 1 in]
        n95 = Concatenate Strings(w350, "-transferfpp-" ("Substring"), w352, ".txt" ("Substring")) -> (w354:string)
        n96 = VISA Write(VISA resource name=w319, write buffer=":PAGE:CHAN:MODE SWE;" ("write buffer (\"\")"), error in (no error)=w318) -> (VISA resource name out=w316:refnum<visa-resource-name>, error out=w317:errorcluster)  [unwired: 1 out]
        n97 = String To Path(string=w354) -> (path=w349:path)
        n98 = case shown="\"d\", Default" w340 {
          tunnel: [w365 w366] -> w338
          frame "s" {
            w365 = u16 0 items=["Single", "Double"] ("sweep mode")
          }
          frame "d", Default {
            w366 = u16 1 items=["Single", "Double"] ("sweep mode")
          }
        }
        n99 = Fract/Exp String To Number(string=w339) -> (number=w323:dbl[])  [unwired: 3 in, 1 out]
        n100 = Index Array(array=w323, index #1=0 ("Index")) -> (element #1=w337:dbl, element #2=w336:dbl, element #3=w335:dbl)  [unwired: 2 in]
        n101 = Delete From Array(array=w323, length=3 ("Length"), index=0 ("Index")) -> (array with subset deleted=w321:dbl[])  [unwired: 1 out]
        n102 = Bundle By Name(cluster=w329, "Gate Start"=w337, "Gate Stop"=w336, "Gate Step (linear only)"=w335, "Gate Compliance"=w347, "Range mode"=w312, "Range"=w311) -> (w313:T3)
        n103 = Index Array(array=w321, index #1=0 ("Index")) -> (element #1=w332:dbl, element #2=w331:dbl, element #3=w330:dbl)  [unwired: 2 in]
        n104 = call <vilib>:"compatOverwrite.vi"("overwrite (F)"=TRUE) -> ("overwrite?"=w299:T7)
        n105 = Bundle By Name(cluster=w328, "Drain Start"=w332, "Drain Stop"=w331, "Drain Step"=w330, "Drain Compliance"=w348, "Range mode"=w310, "Range"=w309) -> (w314:T4)
        n106 = call <userlib>:"4155C Transfer-FPP.vi"("VISA resource name in"=w316, "Gate"=w313, "Drain"=w314, "Timings"=w346, "error in (no error)"=w317, "sweep mode"=w338, "Panel Controls"=w364) -> ("VG"=w355:dbl[], "Outparams"=w307:T8, "VISA Resource Name out"=w344:refnum<visa-resource-name>, "Vprobe2"=w303:dbl[], "ID"=w302:dbl[], "IG"=w301:dbl[], "Vprobe1"=w300:dbl[], "error out"=w345:errorcluster)  [unwired: 13 in]
        n107 = Unbundle By Name(w307) -> ("V2 Step"=w306:dbl, "V2 Start"=w305:dbl, "Number of points"=w304:i32)
        n108 = Open/Create/Replace File(file path (use dialog)=w349, error in=w345, operation (0:open)=w299) -> (refnum out=w361:refnum<file>, error out=w362:errorcluster)  [unwired: 3 in, 1 out]
        n109 = call <userlib>:"4155C Make Big 2d array FPP.vi"("1D Var1"=w355, "1d ID"=w302, "1d Vp2"=w303, "1d IG"=w301, "1d Vp1"=w300, "VAR2 START"=w305, "Number of VAR2 steps"=w304, "VAR2 STEP"=w306, "VAR1 Name"="Vg", "Decimal places in header"=i8 1, "VAR2 Name"="Vd") -> ("Header array"=w357:string[], "Data array"=w358:dbl[][])  [unwired: 15 in]
        n110 = call <userlib>:"4155C Write array to file.vi"("Byte Stream File Refnum"=w361, "Header"=w357, "Data Array"=w358, "error in (no error)"=w362) -> ("dup refnum"=w359:refnum<file>, "error out"=w360:errorcluster)  [unwired: 1 in]
        n111 = Close File(refnum=w359, error in=w360) -> (error out=w343:errorcluster)  [unwired: 1 out]
      }
      frame "output" {
        n112 = Number To Decimal String(number=w416) -> (decimal integer string=w417:string)  [unwired: 1 in]
        n113 = Bundle By Name(cluster=w392, "Emergency Stop"=w424) -> (w434:T6)
        n114 = Delete From Array(array=w407, index=0 ("Index")) -> (deleted portion=w405:string, array with subset deleted=w404:string[])  [unwired: 1 in]
        n115 = Concatenate Strings(w415, "-output-" ("Substring"), w417, ".txt" ("Substring")) -> (w419:string)
        n116 = VISA Write(VISA resource name=w383, write buffer=":PAGE:CHAN:MODE SWE;" ("write buffer (\"\")"), error in (no error)=w380) -> (VISA resource name out=w382:refnum<visa-resource-name>, error out=w381:errorcluster)  [unwired: 1 out]
        n117 = String To Path(string=w419) -> (path=w414:path)
        n118 = case shown="\"d\", Default" w405 {
          tunnel: [w435 w436] -> w403
          frame "s" {
            w435 = u16 0 items=["Single", "Double"] ("sweep mode")
          }
          frame "d", Default {
            w436 = u16 1 items=["Single", "Double"] ("sweep mode")
          }
        }
        n119 = Fract/Exp String To Number(string=w404) -> (number=w386:dbl[])  [unwired: 3 in, 1 out]
        n120 = Index Array(array=w386, index #1=0 ("Index")) -> (element #1=w402:dbl, element #2=w401:dbl, element #3=w400:dbl)  [unwired: 2 in]
        n121 = Delete From Array(array=w386, length=3 ("Length"), index=0 ("Index")) -> (array with subset deleted=w385:dbl[])  [unwired: 1 out]
        n122 = Bundle By Name(cluster=w394, "Gate Start"=w402, "Gate Stop"=w401, "Gate Step (linear only)"=w400, "Gate Compliance"=w412, "Range mode"=w378, "Range"=w377) -> (w433:T3)
        n123 = Index Array(array=w385, index #1=0 ("Index")) -> (element #1=w397:dbl, element #2=w396:dbl, element #3=w395:dbl)  [unwired: 2 in]
        n124 = call <vilib>:"compatOverwrite.vi"("overwrite (F)"=TRUE) -> ("overwrite?"=w368:T7)
        n125 = Bundle By Name(cluster=w393, "Drain Start"=w397, "Drain Stop"=w396, "Drain Step"=w395, "Drain Compliance"=w413, "Range mode"=w376, "Range"=w379) -> (w432:T4)
        n126 = call <userlib>:"4155C Output.vi"("VISA resource name in"=w382, "Gate"=w433, "Drain"=w432, "Timings"=w411, "error in (no error)"=w381, "SMU4"=w370, "sweep mode"=w403, "Panel controls"=w434) -> ("VD"=w420:dbl[], "Outparams"=w373:T8, "VISA Resource Name out"=w409:refnum<visa-resource-name>, "IS"=w423:dbl[], "ID"=w422:dbl[], "IG"=w421:dbl[], "error out"=w410:errorcluster, "SMU4"=w369:dbl[])  [unwired: 12 in]
        n127 = Unbundle By Name(w373) -> ("V2 Step"=w374:dbl, "V2 Start"=w372:dbl, "Number of points"=w371:i32)
        n128 = Open/Create/Replace File(file path (use dialog)=w414, error in=w410, operation (0:open)=w368) -> (refnum out=w429:refnum<file>, error out=w430:errorcluster)  [unwired: 3 in, 1 out]
        n129 = call <userlib>:"4155C Make Big 2d array.vi"("1D Var1"=w420, "1d IS"=w423, "1d ID"=w422, "1d IG"=w421, "1d SMU4"=w369, "SMU4"=w370, "VAR2 START"=w372, "Number of VAR2 steps"=w371, "VAR2 STEP"=w374, "VAR1 Name"="Vd", "Decimal places in header"=i8 1, "VAR2 Name"="Vg") -> ("Header array"=w425:string[], "Data array"=w426:dbl[][])  [unwired: 14 in]
        n130 = call <userlib>:"4155C Write array to file.vi"("Byte Stream File Refnum"=w429, "Header"=w425, "Data Array"=w426, "error in (no error)"=w430) -> ("dup refnum"=w427:refnum<file>, "error out"=w428:errorcluster)  [unwired: 1 in]
        n131 = Close File(refnum=w427, error in=w428) -> (error out=w408:errorcluster)  [unwired: 1 out]
      }
      frame "output-fpp" {
        n132 = Number To Decimal String(number=w489) -> (decimal integer string=w490:string)  [unwired: 1 in]
        n133 = Bundle By Name(cluster=w465, "Emergency Stop"=w493) -> (w503:T6)
        n134 = Delete From Array(array=w480, index=0 ("Index")) -> (deleted portion=w478:string, array with subset deleted=w477:string[])  [unwired: 1 in]
        n135 = Concatenate Strings(w488, "-outputfpp-" ("Substring"), w490, ".txt" ("Substring")) -> (w492:string)
        n136 = VISA Write(VISA resource name=w456, write buffer=":PAGE:CHAN:MODE SWE;" ("write buffer (\"\")"), error in (no error)=w453) -> (VISA resource name out=w455:refnum<visa-resource-name>, error out=w454:errorcluster)  [unwired: 1 out]
        n137 = String To Path(string=w492) -> (path=w487:path)
        n138 = case shown="\"d\", Default" w478 {
          tunnel: [w504 w505] -> w476
          frame "s" {
            w504 = u16 0 items=["Single", "Double"] ("sweep mode")
          }
          frame "d", Default {
            w505 = u16 1 items=["Single", "Double"] ("sweep mode")
          }
        }
        n139 = Fract/Exp String To Number(string=w477) -> (number=w459:dbl[])  [unwired: 3 in, 1 out]
        n140 = Index Array(array=w459, index #1=0 ("Index")) -> (element #1=w475:dbl, element #2=w474:dbl, element #3=w473:dbl)  [unwired: 2 in]
        n141 = Delete From Array(array=w459, length=3 ("Length"), index=0 ("Index")) -> (array with subset deleted=w458:dbl[])  [unwired: 1 out]
        n142 = Bundle By Name(cluster=w467, "Gate Start"=w475, "Gate Stop"=w474, "Gate Step (linear only)"=w473, "Gate Compliance"=w485, "Range mode"=w451, "Range"=w450) -> (w502:T3)
        n143 = Index Array(array=w458, index #1=0 ("Index")) -> (element #1=w470:dbl, element #2=w469:dbl, element #3=w468:dbl)  [unwired: 2 in]
        n144 = call <vilib>:"compatOverwrite.vi"("overwrite (F)"=TRUE) -> ("overwrite?"=w438:T7)
        n145 = Bundle By Name(cluster=w466, "Drain Start"=w470, "Drain Stop"=w469, "Drain Step"=w468, "Drain Compliance"=w486, "Range mode"=w449, "Range"=w452) -> (w501:T4)
        n146 = call <userlib>:"4155C Output-FPP.vi"("VISA resource name in"=w455, "Gate"=w502, "Drain"=w501, "Timings"=w484, "error in (no error)"=w454, "sweep mode"=w476, "Panel controls"=w503) -> ("VD"=w443:dbl[], "Outparams"=w446:T8, "VISA Resource Name out"=w482:refnum<visa-resource-name>, "Vprobe2"=w442:dbl[], "ID"=w441:dbl[], "IG"=w440:dbl[], "Vprobe1"=w439:dbl[], "error out"=w483:errorcluster)  [unwired: 13 in]
        n147 = Unbundle By Name(w446) -> ("V2 Step"=w447:dbl, "V2 Start"=w445:dbl, "Number of points"=w444:i32)
        n148 = Open/Create/Replace File(file path (use dialog)=w487, error in=w483, operation (0:open)=w438) -> (refnum out=w498:refnum<file>, error out=w499:errorcluster)  [unwired: 3 in, 1 out]
        n149 = call <userlib>:"4155C Make Big 2d array FPP.vi"("1D Var1"=w443, "1d ID"=w441, "1d Vp2"=w442, "1d IG"=w440, "1d Vp1"=w439, "VAR2 START"=w445, "Number of VAR2 steps"=w444, "VAR2 STEP"=w447, "VAR1 Name"="Vd", "Decimal places in header"=i8 1, "VAR2 Name"="Vg") -> ("Header array"=w494:string[], "Data array"=w495:dbl[][])  [unwired: 15 in]
        n150 = call <userlib>:"4155C Write array to file.vi"("Byte Stream File Refnum"=w498, "Header"=w494, "Data Array"=w495, "error in (no error)"=w499) -> ("dup refnum"=w496:refnum<file>, "error out"=w497:errorcluster)  [unwired: 1 in]
        n151 = Close File(refnum=w496, error in=w497) -> (error out=w481:errorcluster)  [unwired: 1 out]
      }
      frame "itime" {
        n152 = Delete From Array(array=w518, index=0 ("Index")) -> (deleted portion=w519:string)  [unwired: 1 in, 1 out]
        n153 = case shown="\"l\"" w519 {
          tunnel: w517 -> [w523 w525 w528]
          tunnel: [w522 w524 w527] -> w510
          frame "s" {
            w521 = u32 0 items=["short  ", "medium  ", "long  "] ("integration time 2")
            n154 = Bundle By Name(cluster=w523, "integration time"=w521) -> (w522:T5)
          }
          frame "m", Default {
            w526 = u32 1 items=["short  ", "medium  ", "long  "] ("integration time 2")
            n155 = Bundle By Name(cluster=w525, "integration time"=w526) -> (w524:T5)
          }
          frame "l" {
            w529 = u32 2 items=["short  ", "medium  ", "long  "] ("integration time 2")
            n156 = Bundle By Name(cluster=w528, "integration time"=w529) -> (w527:T5)
          }
        }
      }
      frame "pulsed" {
        n157 = Delete From Array(array=w543, index=0 ("Index")) -> (deleted portion=w544:string, array with subset deleted=w531:string[])  [unwired: 1 in]
        n158 = case shown="\"on\", Default" w544 {
          tunnel: w542 -> [w554 w557]
          tunnel: [w553 w556] -> w535
          tunnel: w531 -> [w551 _]
          frame "on", Default {
            w552 = u16 1 items=["Continuous", "Pulsed"] ("sweep method")
            n159 = Fract/Exp String To Number(string=w551) -> (number=w549:dbl[])  [unwired: 3 in, 1 out]
            n160 = Index Array(array=w549, index #1=0 ("Index")) -> (element #1=w548:dbl, element #2=w547:dbl, element #3=w546:dbl)  [unwired: 2 in]
            n161 = Bundle By Name(cluster=w554, "sweep method"=w552, "Pulse period"=w548, "Base voltage"=w547, "Pulse width"=w546) -> (w553:T5)
          }
          frame "off" {
            w555 = u16 0 items=["Continuous", "Pulsed"] ("sweep method")
            n162 = Bundle By Name(cluster=w557, "sweep method"=w555) -> (w556:T5)
          }
        }
      }
      frame "gaterangemode" {
        n163 = Delete From Array(array=w569, index=0 ("Index")) -> (deleted portion=w570:string)  [unwired: 1 in, 1 out]
        n164 = case shown="\"f\"" w570 {
          tunnel: [w572 w573 w574] -> w559
          frame "a", Default {
            w572 = u16 0 items=["Auto", "Limited", "Fixed"] ("Gate Range\nmode 2")
          }
          frame "f" {
            w573 = u16 2 items=["Auto", "Limited", "Fixed"] ("Gate Range\nmode 2")
          }
          frame "l" {
            w574 = u16 1 items=["Auto", "Limited", "Fixed"] ("Gate Range\nmode 2")
          }
        }
      }
      frame "gaterange" {
        (unwired) u8 11 items=["10fA  ", "100fA  ", "1nA  ", "10nA", "100nA", "1uA", "10uA", "100uA", "1mA", "10mA", "100mA", "1A"] ("Gate Range 2")
        n165 = Delete From Array(array=w593, index=0 ("Index")) -> (deleted portion=w583:string)  [unwired: 1 in, 1 out]
        n166 = Scan Value(string=w583, format string="") -> (value=w581:dbl)  [unwired: 1 in, 1 out]
        n167 = Logarithm Base 10(1:w581) -> (0:w580:dbl)
        n168 = Round To Nearest(number=w580) -> (nearest integer value=w579:dbl)
        n169 = Add(x=w579, y=11.0) -> (x+y=w577:dbl)
        n170 = To Unsigned Byte Integer(number=w577) -> (unsigned 8bit integer=w576:u8)
      }
      frame "drainrange" {
        (unwired) u8 11 items=["10fA  ", "100fA  ", "1nA  ", "10nA", "100nA", "1uA", "10uA", "100uA", "1mA", "10mA", "100mA", "1A"] ("Gate Range 2")
        n171 = Delete From Array(array=w613, index=0 ("Index")) -> (deleted portion=w604:string)  [unwired: 1 in, 1 out]
        n172 = Scan Value(string=w604, format string="") -> (value=w602:dbl)  [unwired: 1 in, 1 out]
        n173 = Logarithm Base 10(1:w602) -> (0:w601:dbl)
        n174 = Round To Nearest(number=w601) -> (nearest integer value=w600:dbl)
        n175 = Add(x=w600, y=11.0) -> (x+y=w598:dbl)
        n176 = To Unsigned Byte Integer(number=w598) -> (unsigned 8bit integer=w597:u8)
      }
      frame "drainrangemode" {
        n177 = Delete From Array(array=w626, index=0 ("Index")) -> (deleted portion=w627:string)  [unwired: 1 in, 1 out]
        n178 = case shown="\"f\"" w627 {
          tunnel: [w629 w630 w631] -> w616
          frame "a", Default {
            w629 = u16 0 items=["Auto", "Limited", "Fixed"] ("Gate Range\nmode 2")
          }
          frame "f" {
            w630 = u16 2 items=["Auto", "Limited", "Fixed"] ("Gate Range\nmode 2")
          }
          frame "l" {
            w631 = u16 1 items=["Auto", "Limited", "Fixed"] ("Gate Range\nmode 2")
          }
        }
      }
      frame "Error", Default {
      }
      frame "logfile" {
        n179 = Number To Decimal String(number=w674) -> (decimal integer string=w678:string)  [unwired: 1 in]
        n180 = Concatenate Strings(w676, "logfile" ("Substring"), w678, ".txt" ("Substring")) -> (w673:string)
        n181 = String To Path(string=w673) -> (path=w646:path)
        n182 = Unbundle(w672) -> ("integration time"=w671:u32, "Short/Long integration time"=w670:dbl, "hold time (sec)"=w669:dbl, "delay time (sec)"=w668:dbl, "Step Time (0 disables)"=w667:dbl, "sweep method"=w666:u16, "Pulse period"=w665:dbl, "Base voltage"=w664:dbl, "Pulse width"=w663:dbl)
        n183 = Build Array(w671, w670, w669, w668, w667, w666, w665, w664, w663, w657, w658, w659, w660, w661, w662) -> (w650:dbl[])
        n184 = Insert Into Array(array=dbl[][] [] ("Input Array"), new element=w650) -> (w649:dbl[][])  [unwired: 2 in]
        n185 = call <vilib>:"compatOverwrite.vi"("overwrite (F)"=TRUE) -> ("overwrite?"=w644:T7)
        n186 = Open/Create/Replace File(file path (use dialog)=w646, error in=w648, operation (0:open)=w644) -> (refnum out=w654:refnum<file>, error out=w653:errorcluster)  [unwired: 3 in, 1 out]
        n187 = call <userlib>:"4155C Write array to file.vi"("Byte Stream File Refnum"=w654, "Header"=string[] ["Int Time", "Short/Long Itime", "Hold time", "Delay time", "Step time", "Sweep method", "Pulse period", "Base Voltage", "Pulse width", "Drain compliance", "Gate compliance", "Gate range mode", "Gate range", "S/D range mode", "S/D range"], "Data Array"=w649, "error in (no error)"=w653) -> ("dup refnum"=w656:refnum<file>, "error out"=w655:errorcluster)  [unwired: 1 in]
        n188 = Close File(refnum=w656, error in=w655) -> (error out=w647:errorcluster)  [unwired: 1 out]
      }
      frame "sample" {
        n189 = Number To Decimal String(number=w728) -> (decimal integer string=w727:string)  [unwired: 1 in]
        n190 = Fract/Exp String To Number(string=w724) -> (number=w684:dbl[])  [unwired: 3 in, 1 out]
        n191 = Concatenate Strings(w702, "-sample-" ("Substring"), w727, ".txt" ("Substring")) -> (w725:string)
        n192 = String To Path(string=w725) -> (path=w706:path)
        n193 = Index Array(array=w684, index=0 ("Index")) -> (element=w722:dbl)
        n194 = Index Array(array=w684, index=2 ("Index")) -> (element=w718:dbl)
        n195 = Index Array(array=w684, index=3 ("Index")) -> (element=w687:dbl)
        n196 = Index Array(array=w684, index=4 ("Index")) -> (element=w683:dbl)
        n197 = call <userlib>:"4155C Config Sampling Measurements.vi"("Sampling interval"=w683, "Sample time"=w687, "Display on/off"=TRUE, "Timings"=w693, "Num Points"=w718, "error in (no error)"=w730, "Drain Compliance"=w729, "Gate Compliance"=w703, "VISA session"=w731) -> ("error out"=w732:errorcluster, "dup VISA resource name"=w733:refnum<visa-resource-name>)  [unwired: 1 in]
        n198 = Index Array(array=w684, index=1 ("Index")) -> (element=w719:dbl)
        n199 = call <userlib>:"4155C Take Sample.vi"("Emergency Stop"=w699, "error in (no error)"=w732, "Vd"=w719, "Vg"=w722, "VISA resource name in"=w733) -> ("error out"=w697:errorcluster, "Id"=w735:dbl[], "Ig"=w708:dbl[], "VISA Resource Name out"=w695:refnum<visa-resource-name>, "Is"=w734:dbl[], "Time"=w712:dbl[])  [unwired: 1 in]
        n200 = Insert Into Array(array=dbl[][] [] ("Input Array"), new element=w712) -> (w711:dbl[][])  [unwired: 2 in]
        n201 = Insert Into Array(array=w711, new element=w708) -> (w710:dbl[][])  [unwired: 2 in]
        n202 = Insert Into Array(array=w710, new element=w735) -> (w709:dbl[][])  [unwired: 2 in]
        n203 = VISA Write(VISA resource name=w695, write buffer=":DISP ON" ("write buffer (\"\")"), error in (no error)=w697) -> (VISA resource name out=w694:refnum<visa-resource-name>, error out=w696:errorcluster)  [unwired: 1 out]
        n204 = Insert Into Array(array=w709, new element=w734) -> (w701:dbl[][])  [unwired: 2 in]
        n205 = Transpose 2D Array(2D array=w701) -> (transposed array=w700:dbl[][])
        n206 = call <vilib>:"compatOverwrite.vi"("overwrite (F)"=TRUE) -> ("overwrite?"=w681:T7)
        n207 = Open/Create/Replace File(file path (use dialog)=w706, error in=w696, operation (0:open)=w681) -> (refnum out=w715:refnum<file>, error out=w714:errorcluster)  [unwired: 3 in, 1 out]
        n208 = call <userlib>:"4155C Write array to file.vi"("Byte Stream File Refnum"=w715, "Header"=string[] ["Time /s", "Ig /A", "Id /A", "Is /A"], "Data Array"=w700, "error in (no error)"=w714) -> ("dup refnum"=w717:refnum<file>, "error out"=w716:errorcluster)  [unwired: 1 in]
        n209 = Close File(refnum=w717, error in=w716) -> (error out=w704:errorcluster)  [unwired: 1 out]
      }
      frame "samplei" {
        n210 = Number To Decimal String(number=w787) -> (decimal integer string=w786:string)  [unwired: 1 in]
        n211 = Fract/Exp String To Number(string=w783) -> (number=w749:dbl[])  [unwired: 3 in, 1 out]
        n212 = Concatenate Strings(w765, "-samplei-" ("Substring"), w786, ".txt" ("Substring")) -> (w784:string)
        n213 = String To Path(string=w784) -> (path=w768:path)
        n214 = Index Array(array=w749, index=4 ("Index")) -> (element=w743:dbl)
        n215 = Index Array(array=w749, index=3 ("Index")) -> (element=w744:dbl)
        n216 = Index Array(array=w749, index=1 ("Index")) -> (element=w746:dbl)
        n217 = Index Array(array=w749, index=0 ("Index")) -> (element=w747:dbl)
        n218 = Index Array(array=w749, index=2 ("Index")) -> (element=w745:dbl)
        n219 = call <userlib>:"4155C Config SamplingI Measurements.vi"("Sample time"=w745, "Display on/off"=TRUE, "Timings"=w757, "Num Points"=w746, "error in (no error)"=w789, "Sampling interval"=w744, "VISA session"=w790) -> ("error out"=w791:errorcluster, "dup VISA resource name"=w792:refnum<visa-resource-name>)  [unwired: 3 in]
        n220 = call <userlib>:"4155C Take SampleI.vi"("Emergency Stop"=w762, "error in (no error)"=w791, "Idg 2"=w747, "Vdg compliance 2"=w743, "VISA resource name in"=w792) -> ("error out"=w760:errorcluster, "Idg"=w794:dbl[], "Vdg"=w770:dbl[], "VISA Resource Name out"=w758:refnum<visa-resource-name>, "Is"=w793:dbl[], "Time"=w774:dbl[])  [unwired: 1 in]
        n221 = Insert Into Array(array=dbl[][] [] ("Input Array"), new element=w774) -> (w773:dbl[][])  [unwired: 2 in]
        n222 = Insert Into Array(array=w773, new element=w770) -> (w772:dbl[][])  [unwired: 2 in]
        n223 = Insert Into Array(array=w772, new element=w794) -> (w771:dbl[][])  [unwired: 2 in]
        n224 = VISA Write(VISA resource name=w758, write buffer=":DISP ON" ("write buffer (\"\")"), error in (no error)=w760) -> (VISA resource name out=w742:refnum<visa-resource-name>, error out=w759:errorcluster)  [unwired: 1 out]
        n225 = Insert Into Array(array=w771, new element=w793) -> (w764:dbl[][])  [unwired: 2 in]
        n226 = Transpose 2D Array(2D array=w764) -> (transposed array=w763:dbl[][])
        n227 = call <vilib>:"compatOverwrite.vi"("overwrite (F)"=TRUE) -> ("overwrite?"=w737:T7)
        n228 = Open/Create/Replace File(file path (use dialog)=w768, error in=w759, operation (0:open)=w737) -> (refnum out=w777:refnum<file>, error out=w776:errorcluster)  [unwired: 3 in, 1 out]
        n229 = call <userlib>:"4155C Write array to file.vi"("Byte Stream File Refnum"=w777, "Header"=string[] ["Time /s", "Vdg /V", "Idg /A", "Is /A"], "Data Array"=w763, "error in (no error)"=w776) -> ("dup refnum"=w779:refnum<file>, "error out"=w778:errorcluster)  [unwired: 1 in]
        n230 = Close File(refnum=w779, error in=w778) -> (error out=w740:errorcluster)  [unwired: 1 out]
        n231 = VISA Write(VISA resource name=w742, write buffer=";:PAGE:SCON:STAN OFF;:PAGE:CHAN:VSU2:DIS;" ("write buffer (\"\")"), error in (no error)=w740) -> (VISA resource name out=w738:refnum<visa-resource-name>, error out=w739:errorcluster)  [unwired: 1 out]
      }
      frame "#" {
        n232 = VISA Write(VISA resource name=w800, write buffer=":DISP ON" ("write buffer (\"\")"), error in (no error)=w799) -> (VISA resource name out=w798:refnum<visa-resource-name>, error out=w797:errorcluster)  [unwired: 1 out]
      }
      frame "stressV" {
        n233 = Number To Decimal String(number=w849) -> (decimal integer string=w848:string)  [unwired: 1 in]
        n234 = Fract/Exp String To Number(string=w845) -> (number=w817:dbl[])  [unwired: 3 in, 1 out]
        n235 = Concatenate Strings(w832, "-stressV-" ("Substring"), w848, ".txt" ("Substring")) -> (w846:string)
        n236 = String To Path(string=w846) -> (path=w836:path)
        n237 = Index Array(array=w817, index=3 ("Index")) -> (element=w814:dbl)
        n238 = Index Array(array=w817, index=1 ("Index")) -> (element=w812:dbl)
        n239 = Index Array(array=w817, index=0 ("Index")) -> (element=w811:dbl)
        n240 = Index Array(array=w817, index=4 ("Index")) -> (element=w816:dbl)
        n241 = Index Array(array=w817, index=2 ("Index")) -> (element=w813:dbl)
        n242 = call <userlib>:"4155C Config V Stress.vi"("VISA session"=w852, "ID compliance"=w814, "VD"=w812, "VG"=w811, "IG compliance"=w813, "error in (no error)"=w851, "Display on/off"=TRUE) -> ("dup VISA resource name"=w854:refnum<visa-resource-name>, "error out"=w853:errorcluster)
        n243 = call <userlib>:"4155C Apply Stress.vi"("error in (no error)"=w853, "Duration"=w816, "Emergency Stop"=w831, "VISA resource name in"=w854) -> ("error out"=w829:errorcluster, "VISA Resource Name out"=w827:refnum<visa-resource-name>)
        n244 = VISA Write(VISA resource name=w827, write buffer=":DISP ON" ("write buffer (\"\")"), error in (no error)=w829) -> (VISA resource name out=w826:refnum<visa-resource-name>, error out=w828:errorcluster)  [unwired: 1 out]
        n245 = call <vilib>:"compatOverwrite.vi"("overwrite (F)"=TRUE) -> ("overwrite?"=w810:T7)
        n246 = Open/Create/Replace File(file path (use dialog)=w836, error in=w828, operation (0:open)=w810) -> (refnum out=w839:refnum<file>, error out=w838:errorcluster)  [unwired: 3 in, 1 out]
        n247 = call <userlib>:"4155C Write array to file.vi"("Byte Stream File Refnum"=w839, "Header"=string[] ["V stress completed successfully", ""], "error in (no error)"=w838) -> ("dup refnum"=w841:refnum<file>, "error out"=w840:errorcluster)  [unwired: 2 in]
        n248 = Close File(refnum=w841, error in=w840) -> (error out=w834:errorcluster)  [unwired: 1 out]
      }
      frame "stressI" {
        n249 = Number To Decimal String(number=w891) -> (decimal integer string=w890:string)  [unwired: 1 in]
        n250 = Fract/Exp String To Number(string=w887) -> (number=w861:dbl[])  [unwired: 3 in, 1 out]
        n251 = Concatenate Strings(w874, "-stressI-" ("Substring"), w890, ".txt" ("Substring")) -> (w888:string)
        n252 = String To Path(string=w888) -> (path=w878:path)
        n253 = Index Array(array=w861, index=1 ("Index")) -> (element=w857:dbl)
        n254 = Index Array(array=w861, index=0 ("Index")) -> (element=w858:dbl)
        n255 = call <userlib>:"4155C Config I Stress.vi"("VISA session"=w894, "IDG"=w858, "VDG compliance"=w857, "error in (no error)"=w893, "Display on/off"=TRUE) -> ("dup VISA resource name"=w896:refnum<visa-resource-name>, "error out"=w895:errorcluster)
        n256 = Index Array(array=w861, index=2 ("Index")) -> (element=w859:dbl)
        n257 = call <userlib>:"4155C Apply Stress.vi"("error in (no error)"=w895, "Duration"=w859, "Emergency Stop"=w873, "VISA resource name in"=w896) -> ("error out"=w871:errorcluster, "VISA Resource Name out"=w869:refnum<visa-resource-name>)
        n258 = VISA Write(VISA resource name=w869, write buffer=":DISP ON" ("write buffer (\"\")"), error in (no error)=w871) -> (VISA resource name out=w868:refnum<visa-resource-name>, error out=w870:errorcluster)  [unwired: 1 out]
        n259 = call <vilib>:"compatOverwrite.vi"("overwrite (F)"=TRUE) -> ("overwrite?"=w856:T7)
        n260 = Open/Create/Replace File(file path (use dialog)=w878, error in=w870, operation (0:open)=w856) -> (refnum out=w881:refnum<file>, error out=w880:errorcluster)  [unwired: 3 in, 1 out]
        n261 = call <userlib>:"4155C Write array to file.vi"("Byte Stream File Refnum"=w881, "Header"=string[] ["I stress completed successfully", ""], "error in (no error)"=w880) -> ("dup refnum"=w883:refnum<file>, "error out"=w882:errorcluster)  [unwired: 2 in]
        n262 = Close File(refnum=w883, error in=w882) -> (error out=w876:errorcluster)  [unwired: 1 out]
      }
      frame "vsu2pulse" {
        n263 = Number To Decimal String(number=w931) -> (decimal integer string=w930:string)  [unwired: 1 in]
        n264 = Fract/Exp String To Number(string=w927) -> (number=w902:dbl[])  [unwired: 3 in, 1 out]
        n265 = Concatenate Strings(w915, "-vsu2-" ("Substring"), w930, ".txt" ("Substring")) -> (w928:string)
        n266 = String To Path(string=w928) -> (path=w919:path)
        n267 = Index Array(array=w902, index=1 ("Index")) -> (element=w901:dbl)
        n268 = Index Array(array=w902, index=0 ("Index")) -> (element=w899:dbl)
        n269 = call <userlib>:"4155C Config VSU2 Stress.vi"("error in (no error)"=w933, "VSU2"=w899, "Display on/off"=TRUE, "VISA session"=w934) -> ("error out"=w935:errorcluster, "dup VISA resource name"=w936:refnum<visa-resource-name>)
        n270 = call <userlib>:"4155C Apply Stress.vi"("error in (no error)"=w935, "Duration"=w901, "Emergency Stop"=w914, "VISA resource name in"=w936) -> ("error out"=w912:errorcluster, "VISA Resource Name out"=w910:refnum<visa-resource-name>)
        n271 = VISA Write(VISA resource name=w910, write buffer=":DISP ON" ("write buffer (\"\")"), error in (no error)=w912) -> (VISA resource name out=w909:refnum<visa-resource-name>, error out=w911:errorcluster)  [unwired: 1 out]
        n272 = call <vilib>:"compatOverwrite.vi"("overwrite (F)"=TRUE) -> ("overwrite?"=w898:T7)
        n273 = Open/Create/Replace File(file path (use dialog)=w919, error in=w911, operation (0:open)=w898) -> (refnum out=w922:refnum<file>, error out=w921:errorcluster)  [unwired: 3 in, 1 out]
        n274 = call <userlib>:"4155C Write array to file.vi"("Byte Stream File Refnum"=w922, "Header"=string[] ["VSU2 pulse completed successfully", ""], "error in (no error)"=w921) -> ("dup refnum"=w924:refnum<file>, "error out"=w923:errorcluster)  [unwired: 2 in]
        n275 = Close File(refnum=w924, error in=w923) -> (error out=w917:errorcluster)  [unwired: 1 out]
      }
      frame "sample-fpp" {
        w945 = string[] ["Time /s", "Id VgVd /A", "Ig VgVd /A", "Vp1 VgVd /V", "Vp2 VgVd /V"] ("Header")
        w949 = "%d" ("format string")
        n276 = Number To Decimal String(number=w999) -> (decimal integer string=w998:string)  [unwired: 1 in]
        n277 = Fract/Exp String To Number(string=w995) -> (number=w983:dbl[])  [unwired: 3 in, 1 out]
        n278 = Concatenate Strings(w989, "-samplefpp-" ("Substring"), w998, ".txt" ("Substring")) -> (w996:string)
        n279 = String To Path(string=w996) -> (path=w957:path)
        n280 = Index Array(array=w983, index=0 ("Index")) -> (element=w943:dbl)
        n281 = Index Array(array=w983, index=1 ("Index")) -> (element=w942:dbl)
        n282 = Index Array(array=w983, index=2 ("Index")) -> (element=w991:dbl)
        n283 = Index Array(array=w983, index=3 ("Index")) -> (element=w981:dbl)
        n284 = call <userlib>:"4155C Config Sampling Measurements FPP.vi"("VISA session"=w1002, "Num Points"=w991, "Vg"=w943, "Display on/off"=TRUE, "Gate Compliance"=w990, "Drain Compliance"=w1000, "Standby"="Standby", "error in (no error)"=w1001, "Timings"=w988, "Vd"=w942, "Sample time"=w981) -> ("dup VISA resource name"=w959:refnum<visa-resource-name>, "error out"=w958:errorcluster)  [unwired: 3 in]
        n285 = Number To Decimal String(number=w943) -> (decimal integer string=w969:string)  [unwired: 1 in]
        n286 = call <userlib>:"4155C Take Sample FPP.vi"("VISA resource name in"=w959, "error in (no error)"=w958, "Emergency Stop"=w960) -> ("Time"=w964:dbl[], "Vp1"=w974:dbl[], "VISA Resource Name out"=w940:refnum<visa-resource-name>, "Ig"=w962:dbl[], "Id"=w963:dbl[], "Vp2"=w972:dbl[], "error out"=w961:errorcluster)  [unwired: 10 in]
        n287 = Insert Into Array(array=dbl[][] [] ("Input Array"), new element=w964) -> (w978:dbl[][])  [unwired: 2 in]
        n288 = Number To Decimal String(number=w942) -> (decimal integer string=w967:string)  [unwired: 1 in]
        n289 = Insert Into Array(array=w978, new element=w963) -> (w977:dbl[][])  [unwired: 2 in]
        n290 = Concatenate Strings("(Vg = " ("Substring"), w969, "V, Vd = " ("Substring"), w967, "V)" ("Substring")) -> (w965:string)
        n291 = Insert Into Array(array=w977, new element=w962) -> (w976:dbl[][])  [unwired: 2 in]
        n292 = Insert Into Array(array=w976, new element=w974) -> (w973:dbl[][])  [unwired: 2 in]
        n293 = Insert Into Array(array=w973, new element=w972) -> (w941:dbl[][])  [unwired: 2 in]
        n294 = call <vilib>:"compatOverwrite.vi"("overwrite (F)"=TRUE) -> ("overwrite?"=w938:T7)
        n295 = Open/Create/Replace File(file path (use dialog)=w957, error in=w961, operation (0:open)=w938) -> (refnum out=w954:refnum<file>, error out=w955:errorcluster)  [unwired: 3 in, 1 out]
        n296 = Array To Spreadsheet String(array=w945, 3:w949) -> (spreadsheet string=w951:string)  [unwired: 1 in]
        n297 = Transpose 2D Array(2D array=w941) -> (transposed array=w971:dbl[][])
        n298 = Search and Replace String(replace all?=TRUE ("replace all? (F)"), input string=w951, search string="VgVd", replace string=w965) -> (result string=w947:string)  [unwired: 4 in, 3 out]
        n299 = Spreadsheet String To Array(format string=w949, spreadsheet string=w947, array type (2D Dbl)=w945) -> (array=w946:string[])  [unwired: 1 in]
        n300 = call <userlib>:"4155C Write array to file.vi"("Byte Stream File Refnum"=w954, "Header"=w946, "Data Array"=w971, "error in (no error)"=w955) -> ("dup refnum"=w952:refnum<file>, "error out"=w953:errorcluster)  [unwired: 1 in]
        n301 = Close File(refnum=w952, error in=w953) -> (error out=w939:errorcluster)  [unwired: 1 out]
      }
      frame "resample-fpp" {
        w1013 = string[] ["Time /s", "Id VgVd /A", "Ig VgVd /A", "Vp1 VgVd /V", "Vp2 VgVd /V"] ("Header")
        w1017 = "%d" ("format string")
        n302 = Number To Decimal String(number=w1059) -> (decimal integer string=w1058:string)  [unwired: 1 in]
        n303 = Fract/Exp String To Number(string=w1055) -> (number=w1006:dbl[])  [unwired: 3 in, 1 out]
        n304 = Concatenate Strings(w1051, "-resamplefpp-" ("Substring"), w1058, ".txt" ("Substring")) -> (w1056:string)
        n305 = String To Path(string=w1056) -> (path=w1025:path)
        n306 = Index Array(array=w1006, index=0 ("Index")) -> (element=w1012:dbl)
        n307 = Index Array(array=w1006, index=1 ("Index")) -> (element=w1011:dbl)
        n308 = Number To Decimal String(number=w1012) -> (decimal integer string=w1035:string)  [unwired: 1 in]
        n309 = call <userlib>:"4155C Take Sample FPP.vi"("VISA resource name in"=w1008, "error in (no error)"=w1007, "Emergency Stop"=w1026) -> ("Time"=w1030:dbl[], "Vp1"=w1040:dbl[], "VISA Resource Name out"=w1010:refnum<visa-resource-name>, "Ig"=w1028:dbl[], "Id"=w1029:dbl[], "Vp2"=w1038:dbl[], "error out"=w1027:errorcluster)  [unwired: 10 in]
        n310 = Insert Into Array(array=dbl[][] [] ("Input Array"), new element=w1030) -> (w1044:dbl[][])  [unwired: 2 in]
        n311 = Number To Decimal String(number=w1011) -> (decimal integer string=w1033:string)  [unwired: 1 in]
        n312 = Insert Into Array(array=w1044, new element=w1029) -> (w1043:dbl[][])  [unwired: 2 in]
        n313 = Concatenate Strings("(Vg = " ("Substring"), w1035, "V, Vd = " ("Substring"), w1033, "V)" ("Substring")) -> (w1031:string)
        n314 = Insert Into Array(array=w1043, new element=w1028) -> (w1042:dbl[][])  [unwired: 2 in]
        n315 = Insert Into Array(array=w1042, new element=w1040) -> (w1039:dbl[][])  [unwired: 2 in]
        n316 = Insert Into Array(array=w1039, new element=w1038) -> (w1005:dbl[][])  [unwired: 2 in]
        n317 = call <vilib>:"compatOverwrite.vi"("overwrite (F)"=TRUE) -> ("overwrite?"=w1004:T7)
        n318 = Open/Create/Replace File(file path (use dialog)=w1025, error in=w1027, operation (0:open)=w1004) -> (refnum out=w1022:refnum<file>, error out=w1023:errorcluster)  [unwired: 3 in, 1 out]
        n319 = Array To Spreadsheet String(array=w1013, 3:w1017) -> (spreadsheet string=w1019:string)  [unwired: 1 in]
        n320 = Transpose 2D Array(2D array=w1005) -> (transposed array=w1037:dbl[][])
        n321 = Search and Replace String(replace all?=TRUE ("replace all? (F)"), input string=w1019, search string="VgVd", replace string=w1031) -> (result string=w1015:string)  [unwired: 4 in, 3 out]
        n322 = Spreadsheet String To Array(format string=w1017, spreadsheet string=w1015, array type (2D Dbl)=w1013) -> (array=w1014:string[])  [unwired: 1 in]
        n323 = call <userlib>:"4155C Write array to file.vi"("Byte Stream File Refnum"=w1022, "Header"=w1014, "Data Array"=w1037, "error in (no error)"=w1023) -> ("dup refnum"=w1020:refnum<file>, "error out"=w1021:errorcluster)  [unwired: 1 in]
        n324 = Close File(refnum=w1020, error in=w1021) -> (error out=w1009:errorcluster)  [unwired: 1 out]
      }
    }
    n325 = local write "Lines left to run:"(w47) -> ()
    n326 = Empty String/Path?(string/path=w47) -> (empty?=w83:bool)
    n327 = Not(x=w83) -> (.not. x?=w82:bool)
  }
  "error out" <- w1
